vi "Logging Message Loop.vi"(8 "error in (no error)":errorcluster, 10 "Data Queue":refnum<queue>, 11 "Message Queues":T1) -> (0 "error out":errorcluster)   [LabVIEW 2016, in "Logging.lvlib"]
doc: "The message loop subVI to handle messages pertaining to logging data."
uses:
  Logging.lvlib
  support/Message Queue/All Message Queues.ctl
  support/Message Queue/Message Cluster.ctl
  Logging Configuration.ctl
  Logging State.ctl
  support/Message Queue/Enqueue Message (Single).vi
  <vilib>/Utility/error.llb/Error Cluster From Error Code.vi
  <vilib>/ErrorRing/Error Ring.xnode
  support/Message Queue/Message Queue.lvlib
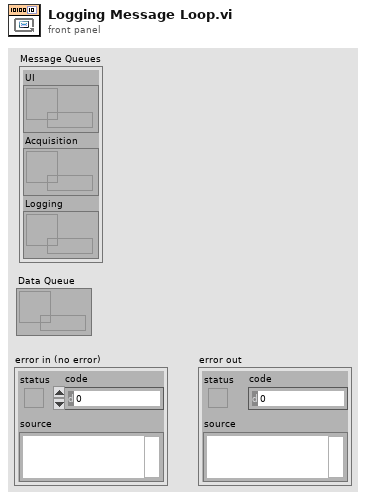
[diagram p1: front panel]
types:
  T1 = typedef "Message Queue.lvlib/All Message Queues.ctl" = cluster{"UI":refnum<queue>, "Acquisition":refnum<queue>, "Logging":refnum<queue>}
  T2 = typedef "Logging.lvlib/Logging Configuration.ctl" = cluster{"Log File Base Path":path, "TDMS File Reference":refnum<k34>, "Enabled":bool, "Disk cache size":u64}
  T3 = typedef "Logging.lvlib/Logging State.ctl" = enum16{"Idle", "Logging"}
  T4 = enum16{"open", "open or create", "create or replace", "create", "open (read-only)"}
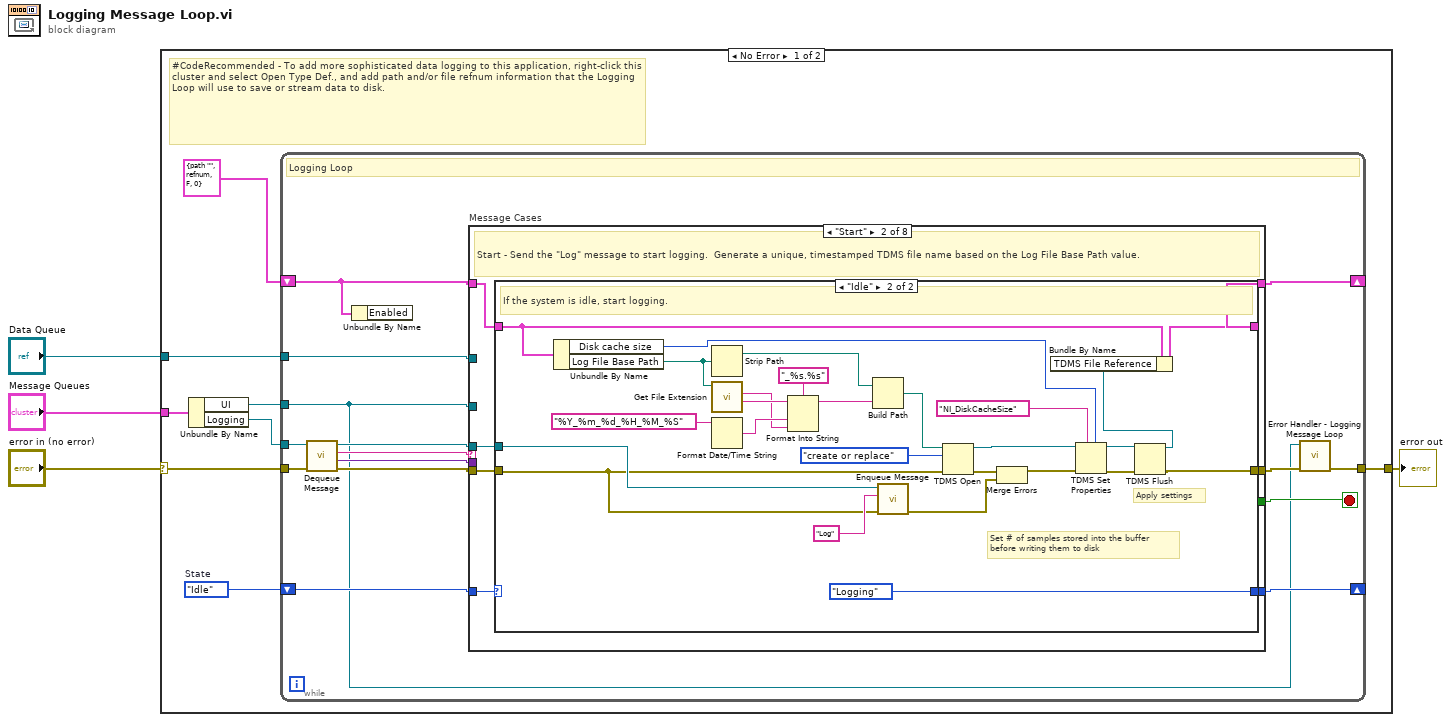
[diagram p0: block diagram]
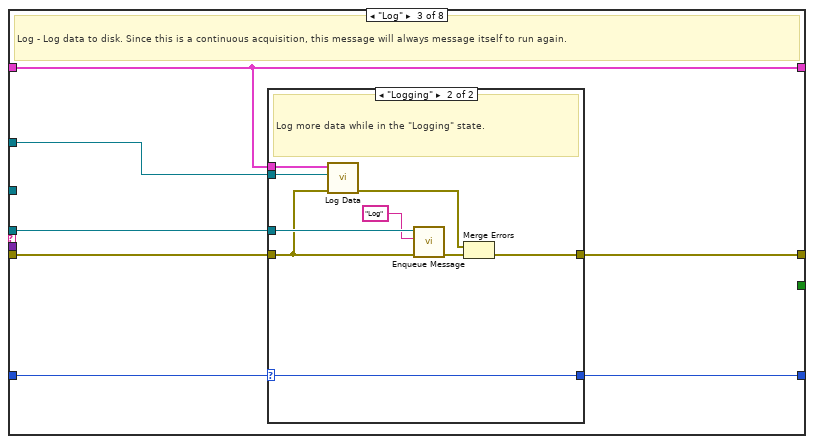
[diagram p4: hidden frame]
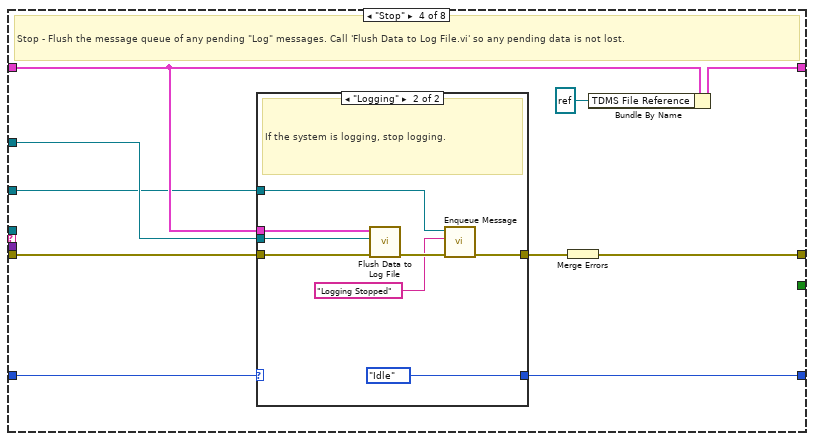
[diagram p6: hidden frame]
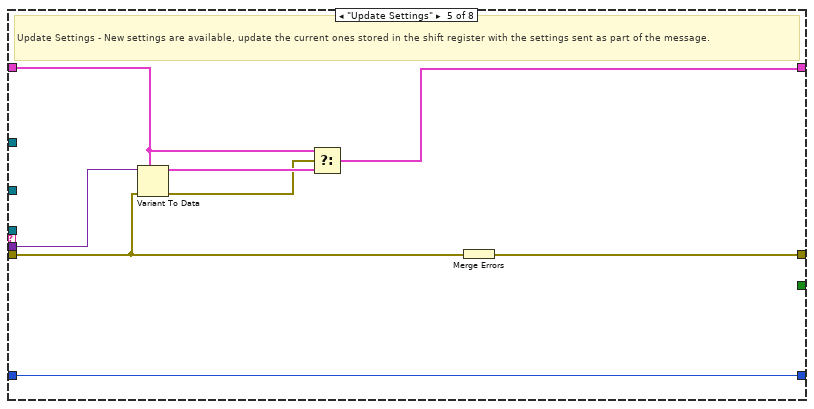
[diagram p8: hidden frame]
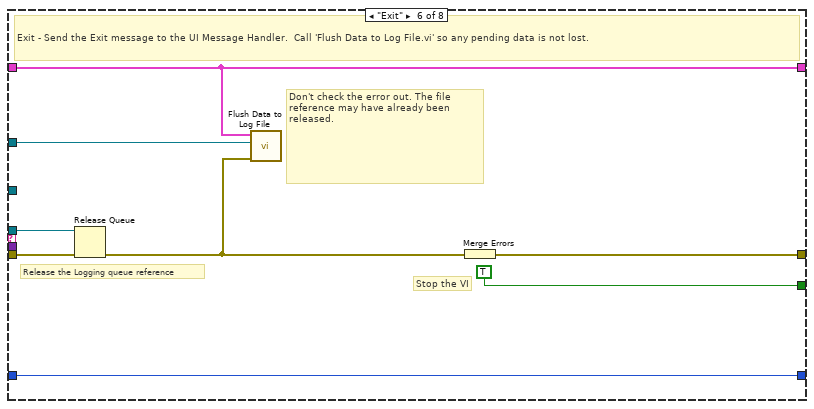
[diagram p9: hidden frame]
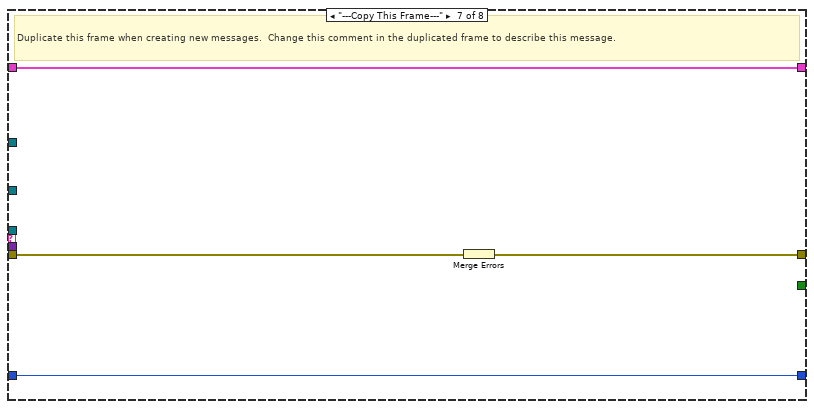
[diagram p10: hidden frame]
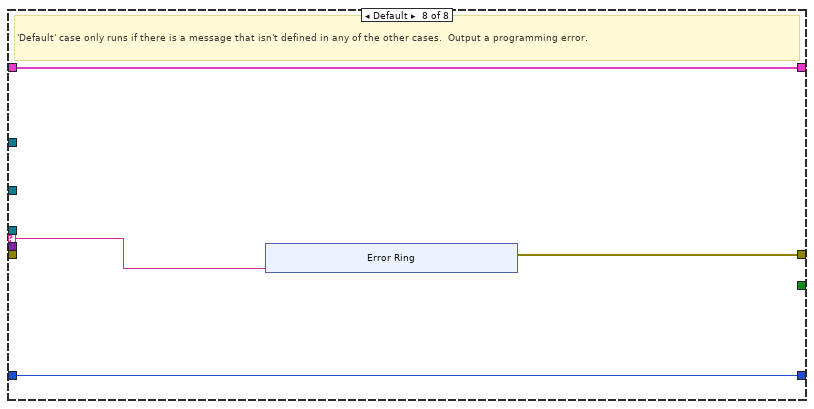
[diagram p11: hidden frame]
diagram:
  n1 = case shown="No Error" "error in (no error)" {
    selector: "error in (no error)" -> [w8 w136]
    tunnel: "Message Queues" -> [w12 _]
    tunnel: [w10 w136] -> w3
    tunnel: "Data Queue" -> [w7 _]
    frame No Error {
      w5 = Logging_State."Idle"  # State
      # "#CodeRecommended - To add more sophisticated data logging to this application, right-click this cluster and select Open Type Def., and add path and/or file refnum information that the Logging Loop will use to save or stream data to disk."
      n2 = Unbundle By Name(w12) -> ("UI"=w6:refnum<queue>, "Logging"=w11:refnum<queue>)
      n3 = while {
        tunnel: w11 -> [w20]
        shift-right: [w27] -> _
        shift-left: T2 {"Log File Base Path"=path "", "TDMS File Reference"=refnum, "Enabled"=FALSE, "Disk cache size"=0} ("Logging Configuration") -> [w13]
        tunnel: w6 -> [w14]
        tunnel: w7 -> [w19]
        shift-right: [w17] -> _
        shift-left: w5 -> [w18]
        tunnel: w8 -> [w25]
        tunnel: [w16] -> w10
        stop <- w26 stop-if-true
        # "Logging Loop"
        n4 = call "Dequeue Message.vi"("error in (no error)"=w25, "Message Queue"=w20) -> ("error out"=w24:errorcluster, "Message Data"=w22:variant, "Message"=w23:string, "dup Message Queue"=w21:refnum<queue>)  [unwired: 6 in]
        n5 = Unbundle By Name(w13) -> ()  [unwired: 1 out]
        n6 = case "Message Cases" shown="\"Start\"" w23 {
          selector: w23 -> [_ _ _ _ _ _ _ w125]
          tunnel: w21 -> [_ w36 w72 _ _ w117 _ _]
          tunnel: w24 -> [w29 w35 w70 w88 w106 w118 w124 _]
          tunnel: [w29 w37 w73 w94 w112 w119 w122 w126] -> w15
          tunnel: w13 -> [w30 w34 w69 w89 w110 w115 w123 w128]
          tunnel: [w30 w33 w69 w92 w107 w115 w123 w128] -> w27
          tunnel: [_ _ _ _ _ TRUE _ _] -> w26
          tunnel: w22 -> [_ _ _ _ w111 _ _ _]
          tunnel: w14 -> [_ _ _ w85 _ _ _ _]
          tunnel: w19 -> [_ _ w71 w90 _ w114 _ _]
          tunnel: w18 -> [w28 w32 w68 w87 w105 w113 w121 w127]
          tunnel: [w28 w31 w67 w86 w105 w113 w121 w127] -> w17
          frame "Initialize" {
            # "Initialize - gets called when first launched. Currently a no-op."
          }
          frame "Start" {
            # "Start - Send the \"Log\" message to start logging.  Generate a unique, timestamped TDMS file name based on the Log File Base Path value."
            n7 = case shown="\"Idle\"" w32 {
              selector: w32 -> [w39 _]
              tunnel: [w38 w43] -> w37
              tunnel: w36 -> [_ w50]
              tunnel: w35 -> [w38 w49]
              tunnel: w34 -> [w40 w51]
              tunnel: [w40 w53] -> w33
              tunnel: [w39 Logging_State."Logging" ("State")] -> w31
              frame "Logging" {
                # "The system is already logging. Ignore the \"Start\" message."
              }
              frame "Idle" {
                # "Apply settings"
                # "Set # of samples stored into the buffer\nbefore writing them to disk"
                # "If the system is idle, start logging."
                n8 = Unbundle By Name(w51) -> ("Disk cache size"=w41:u64, "Log File Base Path"=w65:path)
                n9 = Strip Path(path=w65) -> (stripped path=w62:path)  [unwired: 1 out]
                n10 = call <vilib>:"Get File Extension.vi"("file"=w65) -> ("filename without extension"=w63:string, "lowercase file extension"=w59:string)  [unwired: 6 in, 3 out]
                n11 = Format Date/Time String(time format string (%c)="%Y_%m_%d_%H_%M_%S") -> (date/time string=w60:string)  [unwired: 2 in]
                n12 = Format Into String(format string="_%s.%s", initial string=w63, w60, w59) -> (resulting string=w58:string)  [unwired: 1 in, 1 out]
                n13 = Build Path(base path=w62, name or relative path=w58) -> (appended path=w57:path)
                n14 = call-poly "Enqueue Message.vi"("error in (no error)"=w49, "Message"="Log", "Message Queue"=w50) -> ("error out"=w55:errorcluster)  [unwired: 7 in, 1 out]
                n15 = TDMS Open(8:w49, 10:T4."create or replace" ("operation (0:open)"), 11:w57) -> (0:w56:errorcluster, 3:w48:refnum<k34>)  [unwired: 4 in]
                n16 = Merge Errors(w56, w55) -> (w46:errorcluster)
                n17 = TDMS Set Properties(5:w41, 7:"NI_DiskCacheSize" ("property names"), 8:w46, 11:w48) -> (0:w44:errorcluster, 3:w45:refnum<k34>)  [unwired: 2 in, 2 out]
                n18 = TDMS Flush(4:w44, 7:w45) -> (0:w43:errorcluster, 3:w42:refnum<k34>)
                n19 = Bundle By Name(cluster=w51, "TDMS File Reference"=w42) -> (w53:T2)
              }
            }
          }
          frame "Log" {
            # "Log - Log data to disk. Since this is a continuous acquisition, this message will always message itself to run again."
            n20 = case shown="\"Logging\"" w68 {
              selector: w68 -> [w75 w77]
              tunnel: [w74 w84] -> w73
              tunnel: w72 -> [_ w82]
              tunnel: w71 -> [_ w81]
              tunnel: w70 -> [w74 w76]
              tunnel: w69 -> [_ w78]
              tunnel: [w75 w77] -> w67
              frame "Idle" {
                # "Ignore \"Log\" messages when the logging is idle."
              }
              frame "Logging" {
                # "Log more data while in the \"Logging\" state."
                n21 = call "Log Data.vi"("error in (no error)"=w76, "Data Queue"=w81, "Logging Configuration"=w78) -> ("error out"=w80:errorcluster)  [unwired: 8 in]
                n22 = call-poly "Enqueue Message.vi"("error in (no error)"=w76, "Message"="Log", "Message Queue"=w82) -> ("error out"=w83:errorcluster)  [unwired: 7 in, 1 out]
                n23 = Merge Errors(w80, w83) -> (w84:errorcluster)
              }
            }
          }
          frame "Stop" {
            # "Stop - Flush the message queue of any pending \"Log\" messages. Call 'Flush Data to Log File.vi' so any pending data is not lost."
            n24 = case shown="\"Logging\"" w87 {
              selector: w87 -> [w95 _]
              tunnel: [w96 w99] -> w93
              tunnel: w90 -> [_ w103]
              tunnel: w89 -> [_ w102]
              tunnel: w88 -> [w96 w101]
              tunnel: [w95 Logging_State."Idle" ("State")] -> w86
              tunnel: w85 -> [_ w98]
              frame "Idle" {
                # "The system is already idle. Ignore the \"Stop\" message."
              }
              frame "Logging" {
                # "If the system is logging, stop logging."
                n25 = call "Flush Data to Log File.vi"("error in (no error)"=w101, "Data Queue"=w103, "Logging Configuration"=w102) -> ("error out"=w104:errorcluster)  [unwired: 8 in]
                n26 = call-poly "Enqueue Message.vi"("error in (no error)"=w104, "Message"="Logging Stopped", "Message Queue"=w98) -> ("error out"=w99:errorcluster)  [unwired: 7 in, 1 out]
              }
            }
            n27 = Merge Errors(w93) -> (w94:errorcluster)
            n28 = Bundle By Name(cluster=w89, "TDMS File Reference"=refnum<k34> refnum) -> (w92:T2)
          }
          frame "Update Settings" {
            # "Update Settings - New settings are available, update the current ones stored in the shift register with the settings sent as part of the message."
            n29 = Variant To Data(error in=w106, type=w110, Variant=w111) -> (data=w109:T2, error out=w108:errorcluster)
            n30 = Select(t=w110, s=w108, f=w109) -> (s? t:f=w107:T2)
            n31 = Merge Errors(w106) -> (w112:errorcluster)
          }
          frame "Exit" {
            # "Don't check the error out. The file reference may have already been released."
            # "Release the Logging queue reference"
            # "Stop the VI"
            # "Exit - Send the Exit message to the UI Message Handler.  Call 'Flush Data to Log File.vi' so any pending data is not lost."
            n32 = Release Queue(queue=w117, error in (no error)=w118) -> (error out=w116:errorcluster)  [unwired: 1 in, 2 out]
            n33 = call "Flush Data to Log File.vi"("error in (no error)"=w116, "Data Queue"=w114, "Logging Configuration"=w115) -> ()  [unwired: 8 in, 1 out]
            n34 = Merge Errors(w116) -> (w119:errorcluster)
          }
          frame "---Copy This Frame---" {
            # "Duplicate this frame when creating new messages.  Change this comment in the duplicated frame to describe this message."
            n35 = Merge Errors(w124) -> (w122:errorcluster)
          }
          frame Default {
            # "'Default' case only runs if there is a message that isn't defined in any of the other cases.  Output a programming error."
            n36 = xnode "Error Ring"("parameter 0"=w125) -> ("error out"=w126:errorcluster)
          }
        }
        n37 = call "Error Handler - Logging Message Loop.vi"("error in (no error)"=w15, "Message Queue"=w14) -> ("dup error in"=w16:errorcluster)  [unwired: 8 in, 1 out]
      }
    }
    frame Error {
    }
  }
  "error out" <- w3
